vi "Get Display Text.vi"(8 "error in (no error)":errorcluster, 11 "Element in":refnum<class "Element.lvclass">) -> (0 "error out":errorcluster, 1 "Detail Text":string, 2 "Display Name":string, 3 "Element out":refnum<class "Element.lvclass">)   [LabVIEW 2026, in "VILab.lvlib" / "Element.lvclass"]
uses:
  Element.lvclass
  Element.lvclass/Element.ctl
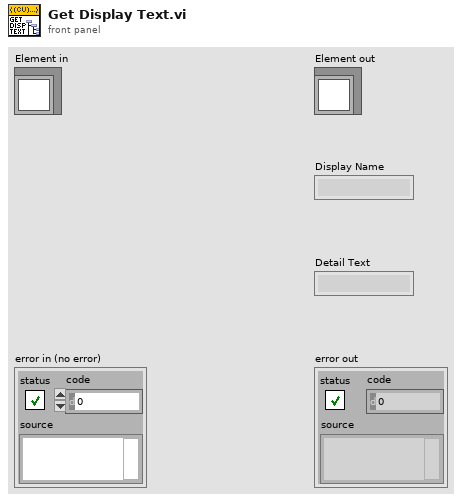
[diagram p1: front panel]
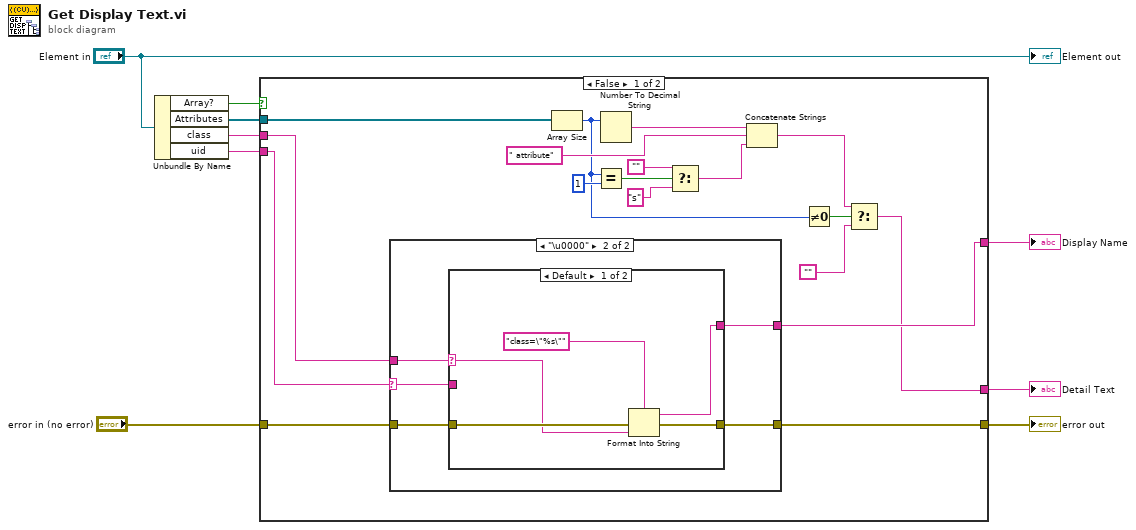
[diagram p0: block diagram]
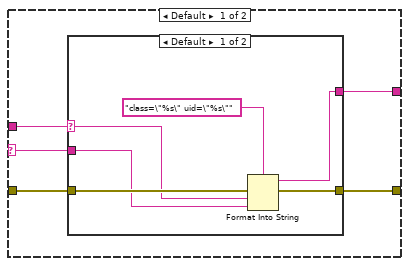
[diagram p2: hidden frame]
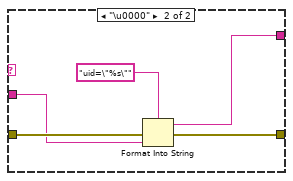
[diagram p3: hidden frame]
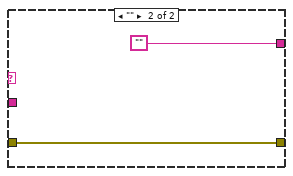
[diagram p4: hidden frame]
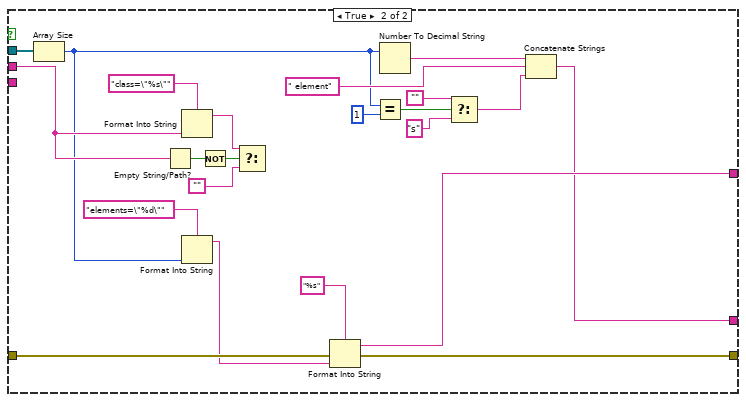
[diagram p5: hidden frame]
diagram:
  n1 = Unbundle By Name("Element in") -> ("Array?"=w1:bool, "Attributes"=w2:refnum<class "Attribute.lvclass">[], "class"=w7:string, "uid"=w6:string)
  n2 = case shown="False" w1 {
    tunnel: w7 -> [w10 w61]
    tunnel: w6 -> [w11 _]
    tunnel: "error in (no error)" -> [w27 w77]
    tunnel: [w26 w76] -> w8
    tunnel: [w17 w74] -> w5
    tunnel: [w12 w66] -> w3
    tunnel: w2 -> [w18 w65]
    frame False {
      n3 = case shown="\"\"" w11 {
        selector: w11 -> [w28 w44]
        tunnel: w27 -> [w32 w48]
        tunnel: [w31 w47] -> w26
        tunnel: [w30 w46] -> w17
        tunnel: w10 -> [w29 w45]
        frame Default {
          n4 = case shown="Default" w29 {
            selector: w29 -> [w35 _]
            tunnel: w32 -> [w38 w43]
            tunnel: [w37 w42] -> w31
            tunnel: [w33 w39] -> w30
            tunnel: w28 -> [w34 w40]
            frame Default {
              n5 = Format Into String(format string="class=\"%s\" uid=\"%s\"", error in=w38, w35, w34) -> (resulting string=w33:string, error out=w37:errorcluster)  [unwired: 1 in]
            }
            frame "\u0000" {
              n6 = Format Into String(format string="uid=\"%s\"", error in=w43, w40) -> (resulting string=w39:string, error out=w42:errorcluster)  [unwired: 1 in]
            }
          }
        }
        frame "\u0000" {
          n7 = case shown="Default" w45 {
            selector: w45 -> [w50 _]
            tunnel: w48 -> [w53 w55]
            tunnel: [w52 w55] -> w47
            tunnel: [w49 ""] -> w46
            tunnel: w44 -> [_ _]
            frame Default {
              n8 = Format Into String(format string="class=\"%s\"", error in=w53, w50) -> (resulting string=w49:string, error out=w52:errorcluster)  [unwired: 1 in]
            }
            frame "" {
            }
          }
        }
      }
      n9 = Array Size(array=w18) -> (size(s)=w16:i32)
      n10 = Equal?(x=w16, y=1) -> (x = y?=w23:bool)
      n11 = Number To Decimal String(number=w16) -> (decimal integer string=w25:string)  [unwired: 1 in]
      n12 = Select(t="", s=w23, f="s") -> (s? t:f=w19:string)
      n13 = Concatenate Strings(w25, " attribute", w19) -> (w14:string)
      n14 = Not Equal To 0?(x=w16) -> (x != 0?=w15:bool)
      n15 = Select(t=w14, s=w15, f="") -> (s? t:f=w12:string)
    }
    frame True {
      n16 = Array Size(array=w65) -> (size(s)=w57:i32)
      n17 = Empty String/Path?(string/path=w61) -> (empty?=w63:bool)
      n18 = Format Into String(format string="class=\"%s\"", w61) -> (resulting string=w60:string)  [unwired: 2 in, 1 out]
      n19 = Format Into String(format string="elements=\"%d\"", w57) -> (resulting string=w56:string)  [unwired: 2 in, 1 out]
      n20 = Not(x=w63) -> (.not. x?=w62:bool)
      n21 = Select(t=w60, s=w62, f="") -> ()  [unwired: 1 out]
      n22 = Format Into String(format string="%s", error in=w77, w56) -> (resulting string=w74:string, error out=w76:errorcluster)  [unwired: 1 in]
      n23 = Equal?(x=w57, y=1) -> (x = y?=w71:bool)
      n24 = Number To Decimal String(number=w57) -> (decimal integer string=w73:string)  [unwired: 1 in]
      n25 = Select(t="", s=w71, f="s") -> (s? t:f=w67:string)
      n26 = Concatenate Strings(w73, " element", w67) -> (w66:string)
    }
  }
  "error out" <- w8
  "Detail Text" <- w3
  "Display Name" <- w5
  "Element out" <- "Element in"
